vi "SECoP_dataModifyStatus.vi"(6 "status text":string, 7 "status code":i64=100, 8 "error in (no error)":errorcluster, 10 "SECoP_dataPtr (in)":T1 {"ptr64" format="%.0x"; "ptr32" format="%.0x"}, 11 "DLL path (in)":T2) -> (0 "error out":errorcluster, 2 "SECoP_dataPtr (out)":T1 {"ptr64" format="%.0x"; "ptr32" format="%.0x"}, 3 "DLL path (out)":T2)   [LabVIEW 2015, in "SECoP.lvlib"]
doc: "Call <b>\"SECoP_dataModifyStatus.vi\"</b> to change the SECoP status value (enum value plus text of SECoP_dataPtr).\n\n<b>DLL path</b> input and output of cluster from \"SECoP-Initialize.vi\"\n<b>SECoP_dataPtr</b> data to access\n<b>status code</b> SECoP status value (0...999)\n<b>status text</b> human readable status text"
uses:
  SECoP.lvlib
  SECoP-libraries.ctl
  SECoP-data.ctl
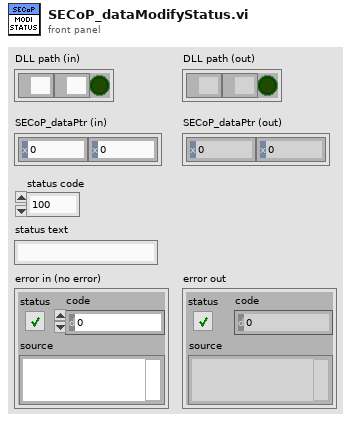
[diagram p1: front panel]
types:
  T1 = typedef "SECoP.lvlib/SECoP-data.ctl" = cluster{"ptr32":u32, "ptr64":u64}
  T2 = typedef "SECoP.lvlib/SECoP-libraries.ctl" = cluster{"serverDLL":path, "variantDLL":path, "cleanup_mode":bool}
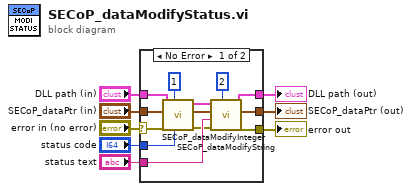
[diagram p0: block diagram]
diagram:
  n1 = case shown="No Error" "error in (no error)" {
    selector: "error in (no error)" -> [w18 w20]
    tunnel: [w15 w22] -> w2
    tunnel: "DLL path (in)" -> [w17 w22]
    tunnel: [w14 w21] -> w3
    tunnel: "SECoP_dataPtr (in)" -> [w14 w21]
    tunnel: "status code" -> [w13 _]
    tunnel: "status text" -> [w12 _]
    tunnel: [w19 w20] -> w1
    frame No Error {
      n2 = call "SECoP_dataModifyInteger.vi"("Value"=w13, "Position"=u32 1, "error in (no error)"=w18, "SECoP_data"=w14, "DLL path (in)"=w17) -> ("error out"=w9:errorcluster, "DLL path (out)"=w16:T2)  [unwired: 5 in]
      n3 = call "SECoP_dataModifyString.vi"("Position"=u32 2, "error in (no error)"=w9, "Value"=w12, "SECoP_dataPtr"=w14, "DLL path (in)"=w16) -> ("error out"=w19:errorcluster, "DLL path (out)"=w15:T2)  [unwired: 5 in]
    }
    frame Error {
    }
  }
  "DLL path (out)" <- w2
  "error out" <- w1
  "SECoP_dataPtr (out)" <- w3
